vi "Open FPGA Reference.vi"(0 "FPGA Resource":T1, 11 "error in":errorcluster) -> (4 "FPGA VI Reference Out":refnum<k20>, 15 "error out":errorcluster)   [LabVIEW 2016, in "Aurora Stream (NI 6592R) (Host).lvlib"]
doc: "Opens a reference to the FPGA Resource.\n\n<B>Input Parameters</B>\n\n<B>FPGA Resource</B> is the FPGA resource to open a reference on.\n\n<B>Output Parameters</B>\n\n<B>FPGA VI Reference Out</B> is a reference to the FPGA on which to perform operations.\n\n<B>error out</B> contains error information. This output provides standard error out functionality."
uses:
  Aurora Stream (NI 6592R) (Host).lvlib
  <vilib>/userdefined/Silver/nirio_resource_slv.ctl
  <vilib>/FPGAPlugInAG/PXIe-6592R/niLvFpga_Open_PXIe-6592R.vi
  <vilib>/rvi/interface/common/dynamic/niFpgaDynamicAddResources.vi
  <vilib>/rvi/interface/nirviOpenFPGA/nirviOpenFPGA.xnode
  FPGA Bitfiles/Stream Controller (NI 6592R).lvbitx
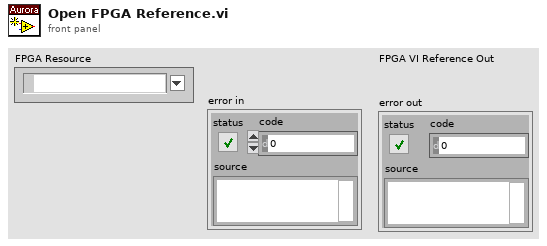
[diagram p1: front panel]
types:
  T1 = typedef "nirio_resource_slv.ctl" = tag
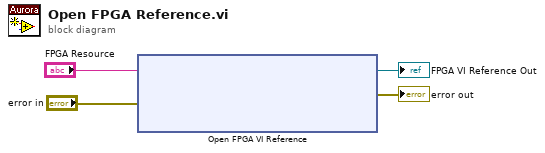
[diagram p0: block diagram]
diagram:
  n1 = xnode "Open FPGA VI Reference"("error in"="error in", "resource name"="FPGA Resource") -> ("FPGA VI Reference Out"=→"FPGA VI Reference Out":refnum<k20>, "error out"=→"error out":errorcluster)
